vi "LinxSpiSetBitOrder.vi"(8 "Error In":errorcluster, 10 "SPI Channel":u8, 11 "LINX Resource":T1) -> (0 "Error Out":errorcluster, 3 "LINX Resource":T1)   [LabVIEW 2014, in "LMH-LINX.lvlib" / "Local IO.lvlib"]
uses:
  <vilib>/MakerHub/LINX/Private/Local IO/Local IO.lvlib
  <vilib>/MakerHub/LINX/Private/Type Defs/LINX Ref.ctl
  <vilib>/MakerHub/LINX/Private/Type Defs/Platform.ctl
  <vilib>/MakerHub/LINX/Private/Type Defs/Interface.ctl
  <vilib>/MakerHub/LINX/Private/Device/Type Defs/LINX Device Config.ctl
  <vilib>/MakerHub/LINX/Private/Device/Type Defs/TCP Config.ctl
  <vilib>/MakerHub/LINX/Private/Device/Type Defs/Channels.ctl
  <vilib>/MakerHub/LINX/Private/Type Defs/Error Type.ctl
  <vilib>/myRIO/Common/Instrument Driver Framework/myRIO v1.0/SPI/typedefs/SPI Frame Length.ctl
  <vilib>/myRIO/Common/Instrument Driver Framework/myRIO v1.0/SPI/typedefs/SPI Data Direction.ctl
  <vilib>/myRIO/Common/Instrument Driver Framework/myRIO v1.0/SPI/typedefs/SPI Clock Polarity.ctl
  <vilib>/myRIO/Common/Instrument Driver Framework/myRIO v1.0/SPI/typedefs/SPI Clock Phase.ctl
  <vilib>/myRIO/Instrument Drivers/Onboard IO/SPI/typedefs/SPI User Configuration.ctl
  <vilib>/myRIO/Instrument Drivers/Onboard IO/SPI/SPI.lvlib
  <vilib>/MakerHub/LINX/Private/myRIO/myRIO.lvlib
  <vilib>/MakerHub/LINX/LMH-LINX.lvlib
  <vilib>/MakerHub/LINX/Private/Type Defs/Channel FGV States.ctl
  liblinxdevice.dll
  <vilib>/MakerHub/LINX/Private/Device/Device.lvlib
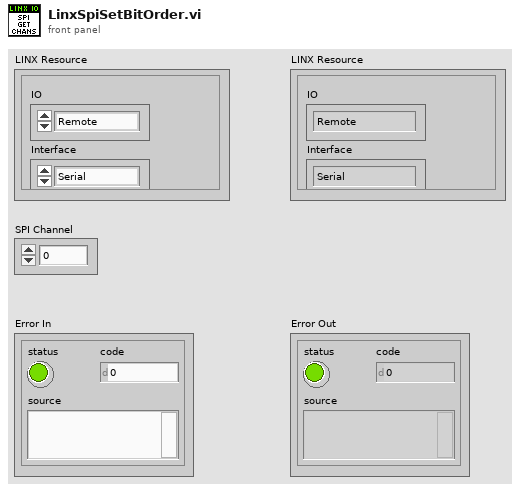
[diagram p1: front panel]
types:
  T1 = typedef "LMH-LINX.lvlib/LINX Ref.ctl" = cluster{"IO":T2, "Interface":T3, "LINX Device Config":T4}
  T2 = typedef "LMH-LINX.lvlib/Platform.ctl" = enum16{"Remote", "Local"}
  T3 = typedef "LMH-LINX.lvlib/Interface.ctl" = enum16{"Serial", "TCP"}
  T4 = typedef "LMH-LINX.lvlib/Device.lvlib/LINX Device Config.ctl" = cluster{"Interface":T3, "COM Port":refnum<visa-resource-name>, "TCP Configuration":T5, "Device Family":u8, "Device ID":u8, "Device Name":string, "TCP Ref":refnum<k5>, "Channels":T6}
  T5 = typedef "LMH-LINX.lvlib/Device.lvlib/TCP Config.ctl" = cluster{"IP Address":string, "Port":u16}
  T6 = typedef "LMH-LINX.lvlib/Channels.ctl" = cluster{"DI":u8[], "DO":u8[], "AI":u8[], "AO":u8[], "PWM":u8[], "QE":u8[], "UART":u8[], "I2C 2":u8[], "SPI":u8[], "CAN":u8[], "Servo":u8[], "AI Ref (V)":dbl, "AI Resolution (Bits)":u8, "AO Ref (V)":dbl, "AO Resolution (Bits)":u8}
  T7 = typedef "LMH-LINX.lvlib/Error Type.ctl" = enum16{"Unknown", "Timeout", "Corrupt Return Packet", "Unable To Connect", "Command Not Supported", "Channel DNE", "Invalid COM Config", "Firmware Version Mismatch", "myRIO Support", "CMD Specific Error", "Local IO Not Supported"}
  T8 = typedef "LMH-LINX.lvlib/Channel FGV States.ctl" = enum16{"Initialize", "Get", "Set"}
  T9 = typedef "SPI.lvlib/SPI User Configuration.ctl" = cluster{"Frequency [Hz]":dbl, "Clock Phase":T10, "Clock Polarity":T11, "Data Direction":T12, "Frame Length":T13}
  T10 = typedef "SPI Clock Phase.ctl" = enum8{"Leading", "Trailing"}
  T11 = typedef "SPI Clock Polarity.ctl" = enum8{"Low", "High"}
  T12 = typedef "SPI Data Direction.ctl" = enum8{"Most significant bit first", "Least significant bit first"}
  T13 = typedef "SPI Frame Length.ctl" = u8
  T14 = typedef "SPI.lvlib/SPI Reference.ctl" = cluster{"myRIO Reference":T15, "SPI Channels Enum":T19, "SPI Configuration":T20}
  T15 = typedef "myRIO Generic Hardware Reference.ctl" = cluster{"myRIO Model":T16, "myRIO Hardware Reference":T17}
  T16 = typedef "Hardware Version Enum.ctl" = enum16{"Unknown", "myRIO-1900", "myRIO-1950"}
  T17 = typedef "myRIO v1.0 Reference.ctl" = cluster{"Generic FPGA Reference":T18, "Allow multiple opens":bool}
  T18 = typedef "Generic FPGA Reference.ctl" = refnum<k20>
  T19 = typedef "SPI Channels Enum.ctl" = enum16{"Not Connected", "A/SPI", "B/SPI"}
  T20 = typedef "SPI.lvlib/SPI Configuration.ctl" = cluster{"Frequency [Hz]":dbl, "Clock Phase":T10, "Clock Polarity":T11, "Data Direction":T12, "Frame Length":T13}
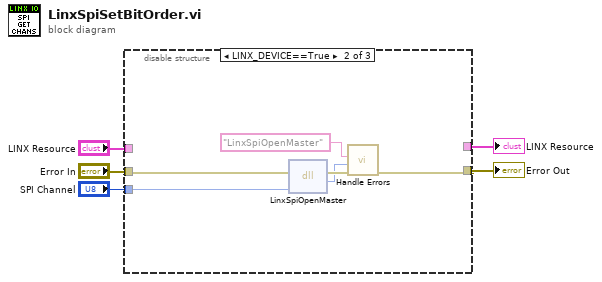
[diagram p0: block diagram]
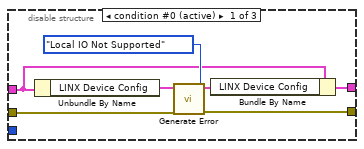
[diagram p2: hidden frame]
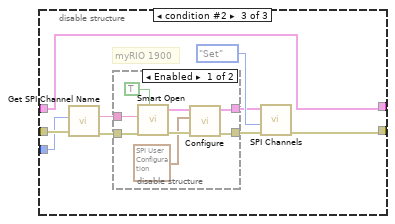
[diagram p3: hidden frame]
diagram:
  n1 = disable-structure shown="LINX_DEVICE==True" {
    disable-tunnel: [w6 _ w19] -> w4
    disable-tunnel: "LINX Resource" -> [w8 _ w19]
    disable-tunnel: "Error In" -> [w11 w15 w22]
    disable-tunnel: [w10 w16 w20] -> w5
    disable-tunnel: "SPI Channel" -> [_ w13 w21]
    frame condition #0 (active) {
      n2 = Unbundle By Name(w8) -> ("LINX Device Config"=w9:T4)
      n3 = call <vilib>:"Generate Error.vi"("Error In"=w11, "Error Type"=Error_Type."Local IO Not Supported", "LINX Device Config"=w9) -> ("Error Out"=w10:errorcluster, "Dup LINX Device Config"=w7:T4)  [unwired: 7 in]
      n4 = Bundle By Name(cluster=w8, "LINX Device Config"=w7) -> (w6:T1)
    }
    frame condition #1 {
      n5 = dll-call lib="liblinxdevice.*" fn="LinxSpiOpenMaster"(error in=w15, "channel"=w13) -> (error out=w17:errorcluster, "Status"=w14:i32)  [unwired: 3 in, 1 out]
      n6 = call <vilib>:"Handle Errors.vi"("Error In"=w17, "LinxStatus"=w14, "Function Name"="LinxSpiOpenMaster") -> ("Error Out"=w16:errorcluster)  [unwired: 7 in, 1 out]
    }
    frame condition #2 {
      # "myRIO 1900"
      n7 = call <vilib>:"Get SPI Channel Name.vi"("Error In"=w22, "SPI Channel"=w21) -> ("Error Out"=w23:errorcluster, "myRIO SPI Channel"=w25:string)  [unwired: 8 in]
      n8 = disable-structure shown="Enabled" {
        disable-tunnel: w23 -> [w34 _]
        disable-tunnel: [w30 _] -> w24
        disable-tunnel: w25 -> [w33 _]
        disable-tunnel: [w29 _] -> w26
        frame Enabled {
          n9 = call <vilib>:"Smart Open.vi"("Allow multiple opens?"=TRUE, "error in (no error)"=w34, "Channel Name"=w33) -> ("error out"=w31:errorcluster, "SPI Ref Out"=w32:T14)  [unwired: 7 in]
          n10 = call <vilib>:"Configure.vi"("error in (no error)"=w31, "SPI User Configuration"=T9 {"Frequency [Hz]"=0.0, "Clock Phase"=enum."Leading", "Clock Polarity"=enum."Low", "Data Direction"=enum."Most significant bit first", "Frame Length"=0}, "SPI Ref In"=w32) -> ("error out"=w30:errorcluster, "SPI Ref Out"=w29:T14)  [unwired: 7 in]
        }
        frame Disabled {
        }
      }
      n11 = call <vilib>:"SPI Channels.vi"("Error In"=w24, "Channel State"=Channel_FGV_States."Set", "SPI Channel"=w26) -> ("Error Out"=w20:errorcluster)  [unwired: 7 in, 1 out]
    }
  }
  "LINX Resource" <- w4
  "Error Out" <- w5
